vi "configure_version.vi"(8 "error in (no error)":errorcluster, 11 "lv-build-default in":refnum<class "lv-builder-default.lvclass">) -> (0 "error out":errorcluster, 3 "lv-build-default out":refnum<class "lv-builder-default.lvclass">)   [LabVIEW 2015, in "lv-builder-default.lvclass"]
uses:
  lv-builder-default.lvclass
  lv-builder-default.lvclass/lv-builder-default.ctl
  lv-builder-default.lvlib
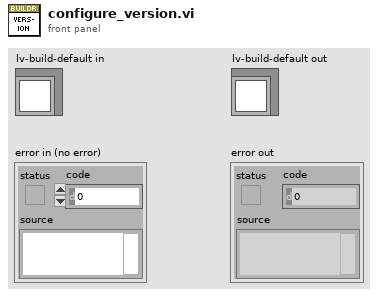
[diagram p1: front panel]
types:
  T1 = typedef "lv-builder-default.lvlib/version.ctl" = cluster{"project_file":string, "major":u32, "minor":u32, "fix":u32, "suffix":string}
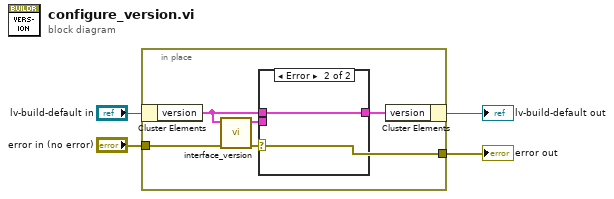
[diagram p0: block diagram]
diagram:
  n1 = in-place {
    in-place-border: "error in (no error)" -> [w9]
    in-place-border: [w8] -> w2
    n2 = in-place-cluster #1("lv-build-default in") -> ("version"=w7:T1)
    n3 = call "interface_version.vi"("error in (no error)"=w9, "version in"=w7) -> ("error out"=w8:errorcluster, "version out"=w6:T1)  [unwired: 8 in]
    n4 = case shown="Error" w8 {
      tunnel: w7 -> [_ w11]
      tunnel: w6 -> [w10 _]
      tunnel: [w10 w11] -> w5
      frame No Error {
      }
      frame Error {
      }
    }
    n5 = in-place-cluster #1("version"=w5) -> (→"lv-build-default out":refnum<class "lv-builder-default.lvclass">)
  }
  "error out" <- w2
